vi "Pad Calibration Summary.vi"(8 "Error In":errorcluster, 10 "device ID":refnum<k1>, 11 "Calibration Cluster":T3) -> (0 "Error Out":errorcluster, 2 "device ID out":refnum<k1>)   [LabVIEW 2014]
uses:
  Controls/Controllers Clusters/Game Pad Calibration Cluster.ctl
  <vilib>/Utility/inputDevices.llb/joystickAcquire.vi
panel:
  out "Motor On":bool
  out "Steering Wheel":i8(slide) min=-100 max=100 scale=-100.0..100.0
  out "Speed":i8(knob) scale=-100.0..100.0
  in  "button info":T1
  in  "axis info":T2
  in  "OK Button":bool
  out "Steering Axis Zero":i32
  out "Steering Axis Max":i32
  out "Steering Axis Number":u8
  out "Back Speed Axis Zero":i32
  out "Back Speed Axis Max":i32
  out "Back Speed Axis Number":u8
  out "Speed Axis Zero":i32
  out "Speed Axis Max":i32
  out "Speed Axis Number":u8
  out "Safety Button Number":u8
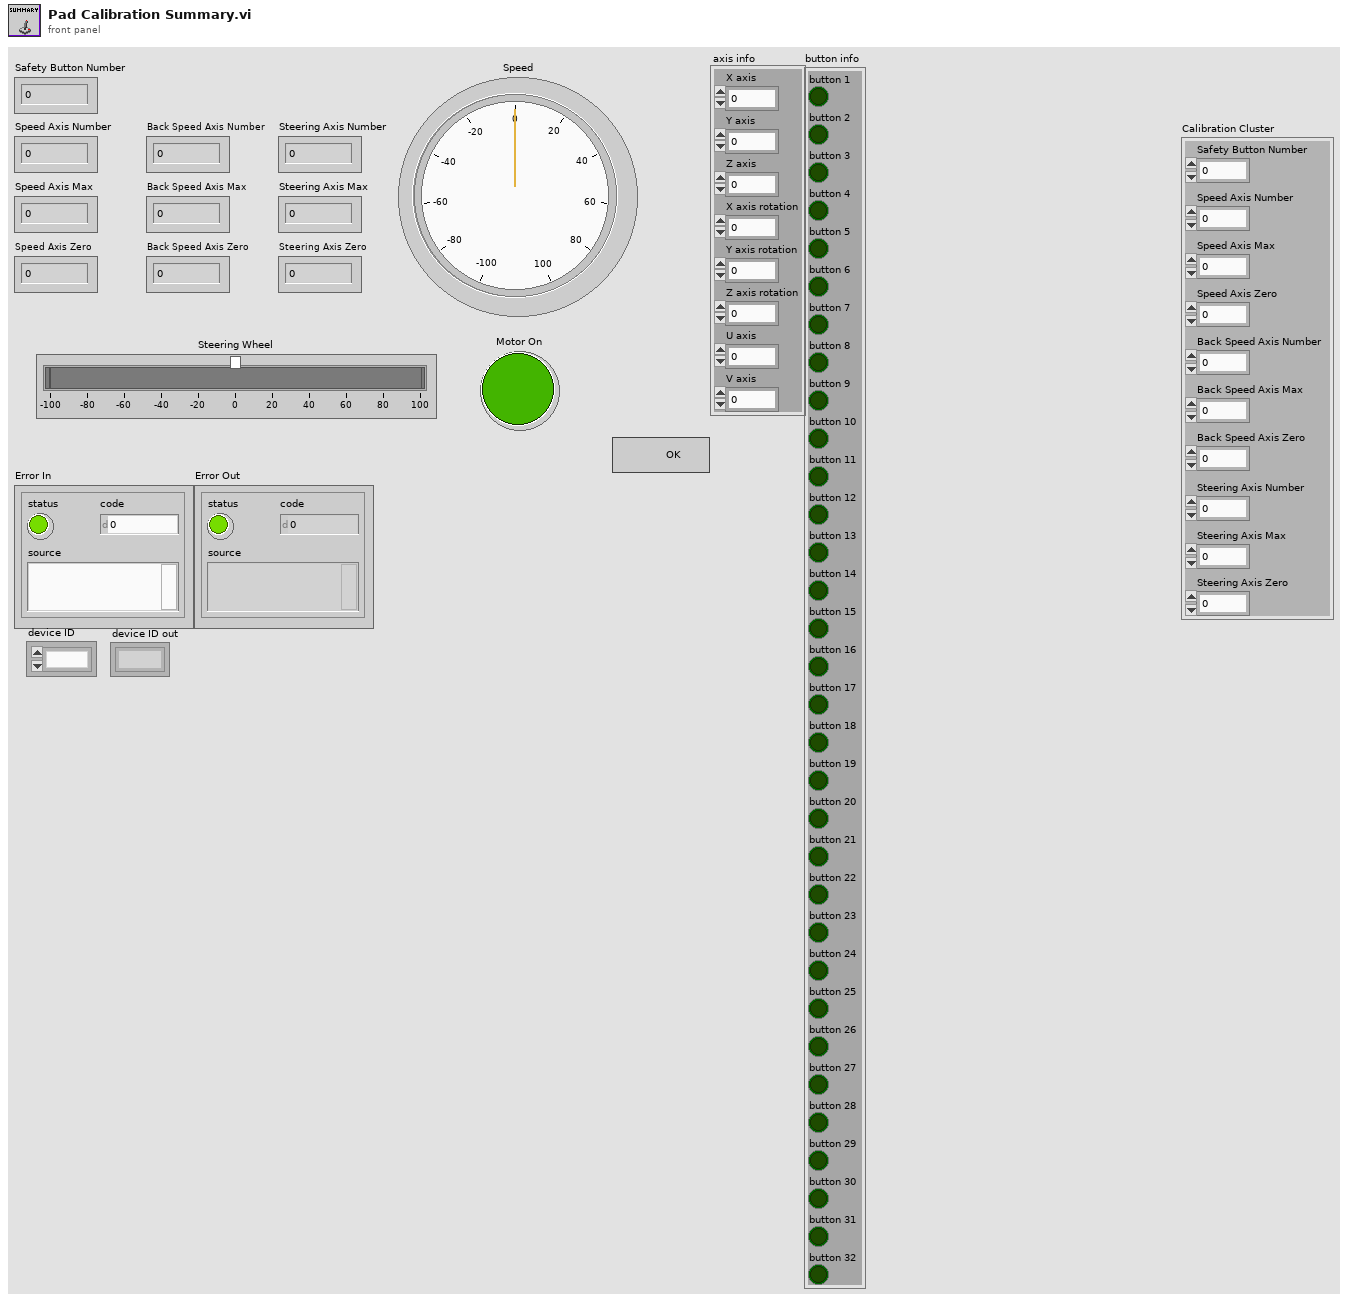
[diagram p1: front panel]
types:
  T1 = cluster{"button 1":bool, "button 2":bool, "button 3":bool, "button 4":bool, "button 5":bool, "button 6":bool, "button 7":bool, "button 8":bool, "button 9":bool, "button 10":bool, "button 11":bool, "button 12":bool, "button 13":bool, "button 14":bool, "button 15":bool, "button 16":bool, "button 17":bool, "button 18":bool, "button 19":bool, "button 20":bool, "button 21":bool, "button 22":bool, "button 23":bool, "button 24":bool, "button 25":bool, "button 26":bool, "button 27":bool, "button 28":bool, "button 29":bool, "button 30":bool, "button 31":bool, "button 32":bool}
  T2 = cluster{"X axis":i32, "Y axis":i32, "Z axis":i32, "X axis rotation":i32, "Y axis rotation":i32, "Z axis rotation":i32, "U axis":i32, "V axis":i32}
  T3 = typedef "Game Pad Calibration Cluster.ctl" = cluster{"Safety Button Number":u8, "Speed Axis Number":u8, "Speed Axis Max":i32, "Speed Axis Zero":i32, "Back Speed Axis Number":u8, "Back Speed Axis Max":i32, "Back Speed Axis Zero":i32, "Steering Axis Number":u8, "Steering Axis Max":i32, "Steering Axis Zero":i32}
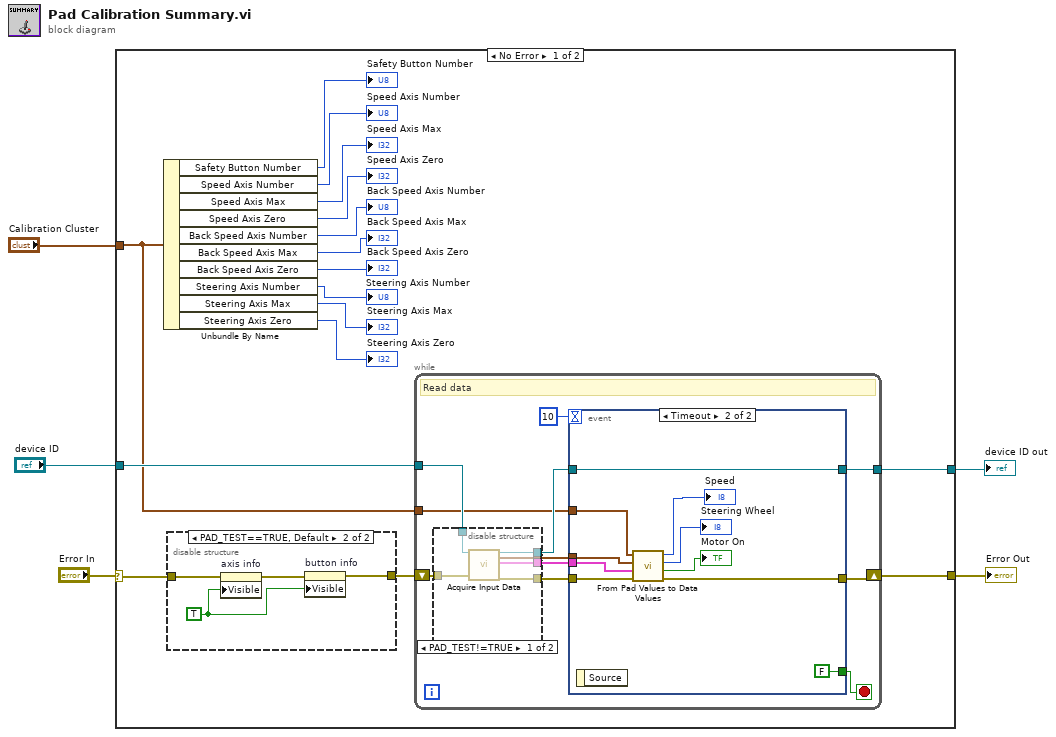
[diagram p0: block diagram]
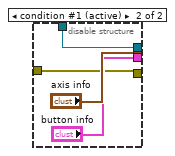
[diagram p2: hidden frame]
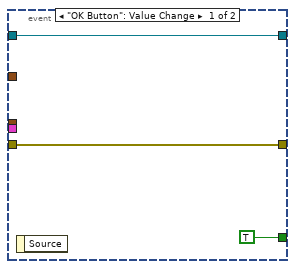
[diagram p3: hidden frame]
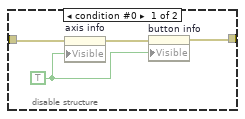
[diagram p4: hidden frame]
diagram:
  n1 = case shown="No Error" "Error In" {
    selector: "Error In" -> [w10 w65]
    tunnel: [w11 w65] -> w4
    tunnel: "Calibration Cluster" -> [w6 _]
    tunnel: "device ID" -> [w8 w64]
    tunnel: [w7 w64] -> w1
    frame No Error {
      n2 = Unbundle By Name(w6) -> ("Safety Button Number"=→"Safety Button Number":u8, "Speed Axis Number"=→"Speed Axis Number":u8, "Speed Axis Max"=→"Speed Axis Max":i32, "Speed Axis Zero"=→"Speed Axis Zero":i32, "Back Speed Axis Number"=→"Back Speed Axis Number":u8, "Back Speed Axis Max"=→"Back Speed Axis Max":i32, "Back Speed Axis Zero"=→"Back Speed Axis Zero":i32, "Steering Axis Number"=→"Steering Axis Number":u8, "Steering Axis Max"=→"Steering Axis Max":i32, "Steering Axis Zero"=→"Steering Axis Zero":i32)
      n3 = disable-structure shown="PAD_TEST==TRUE, Default" {
        disable-tunnel: w10 -> [w58 w63]
        disable-tunnel: [w57 w61] -> w9
        frame condition #0 {
          w56 = TRUE
          n4 = property on="axis info" class="Clust (strict)"(error in=w58, "Visible"=w56) -> (error out=w59:errorcluster)  [unwired: 1 in, 1 out]
          n5 = property on="button info" class="Clust (strict)"(error in=w59, "Visible"=w56) -> (error out=w57:errorcluster)  [unwired: 1 in, 1 out]
        }
        frame condition #1 (active) {
          w60 = TRUE
          n6 = property on="axis info" class="Clust (strict)"(error in=w63, "Visible"=w60) -> (error out=w62:errorcluster)  [unwired: 1 in, 1 out]
          n7 = property on="button info" class="Clust (strict)"(error in=w62, "Visible"=w60) -> (error out=w61:errorcluster)  [unwired: 1 in, 1 out]
        }
      }
      n8 = while {
        shift-right: [w28] -> w11
        shift-left: w9 -> [w30]
        tunnel: w8 -> [w27]
        tunnel: [w26] -> w7
        tunnel: w6 -> [w22]
        stop <- w31 stop-if-true
        # "Read data"
        n9 = disable-structure shown="PAD_TEST!=TRUE" {
          disable-tunnel: w30 -> [w38 w40]
          disable-tunnel: [w37 "axis info"] -> w24
          disable-tunnel: [w36 "button info"] -> w23
          disable-tunnel: [w35 w40] -> w29
          disable-tunnel: w27 -> [w34 w39]
          disable-tunnel: [w33 w39] -> w25
          frame condition #0 {
            n10 = call-poly <vilib>:"Acquire Input Data.vi"("device ID"=w34, "error in (no error)"=w38) -> ("device ID"=w33:refnum<k1>, "axis info"=w37:T2, "button info"=w36:T1, "error out"=w35:errorcluster)  [unwired: 13 in, 1 out]
          }
          frame condition #1 (active) {
          }
        }
        n11 = event shown="[1] Timeout" {
          selector: _ -> [_ _]
          dyn-events: _ -> [_ _]
          timeout: 10 -> [_ _]
          tunnel: [TRUE FALSE] -> w31
          tunnel: w29 -> [w44 w53]
          tunnel: [w44 w47] -> w28
          tunnel: [w43 w54] -> w26
          tunnel: w25 -> [w43 w54]
          tunnel: w24 -> [_ w51]
          tunnel: w23 -> [_ w50]
          tunnel: w22 -> [_ w52]
          event "OK Button": Value Change {
            n12 = event-data() -> ()  [unwired: 1 in, 1 out]
          }
          event Timeout {
            n13 = event-data() -> ()  [unwired: 1 in, 1 out]
            n14 = call "From Pad Values to Data Values.vi"("Error In"=w53, "button info"=w50, "axis info"=w51, "Calibration Cluster"=w52) -> ("Error Out"=w47:errorcluster, "Motor On"=→"Motor On":bool, "Steering Wheel"=→"Steering Wheel":i8, "Speed"=→"Speed":i8)  [unwired: 4 in]
          }
        }
      }
    }
    frame Error {
    }
  }
  "Error Out" <- w4
  "device ID out" <- w1
